vi "Get Provided Interface and Service Class.vi"(8 "error in (no error)":errorcluster, 11 "session factory in":refnum<class "Session Factory.lvclass">) -> (0 "error out":errorcluster, 1 "service class":string, 2 "provided interface":string, 3 "session factory out":refnum<class "Session Factory.lvclass">)   [LabVIEW 2021, in "Keysight 34461A DMM Instrument.lvlib" / "Session Factory.lvclass"]
doc: "Returns the provided interface and service class that will be used to query the NI Discovery Service for the address and port of the instrument's gRPC server. If your instrument does not use a gRPC server then you do not have to override this VI."
uses:
  Session Factory.lvclass
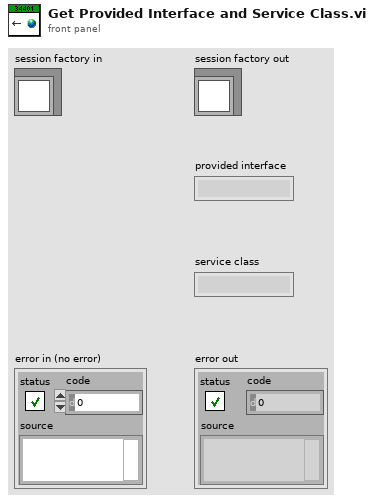
[diagram p1: front panel]
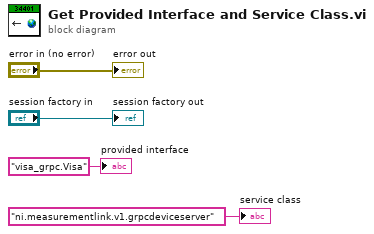
[diagram p0: block diagram]
diagram:
  "error out" <- "error in (no error)"
  "session factory out" <- "session factory in"
  "provided interface" <- "visa_grpc.Visa" ("provided interface")
  "service class" <- "ni.measurementlink.v1.grpcdeviceserver" ("service class")
